vi "Make DIO JSON.vi"(9 "Force":bool, 10 "DIO prev":T1={"type"="DIO", "device"="", "name"="", "data"={"<init"=FALSE, "<>value"=FALSE, "<pulse_length"=0, "<input"=FALSE}}, 11 "DIO new":T1={"type"="DIO", "device"="", "name"="", "data"={"<init"=FALSE, "<>value"=FALSE, "<pulse_length"=0, "<input"=FALSE}}) -> (3 "delta JSON":string)   [LabVIEW 2019]
uses:
  DIO data proto.ctl
  DIO proto.ctl
panel:
  out "Complete JSON":string
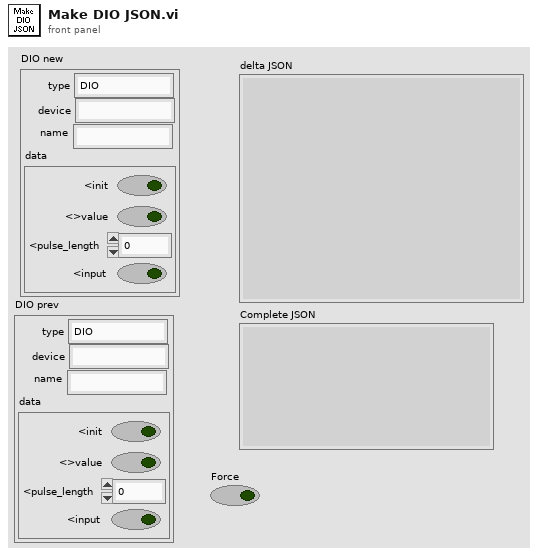
[diagram p1: front panel]
types:
  T1 = typedef "DIO proto.ctl" = cluster{"type":string, "device":string, "name":string, "data":T2}
  T2 = typedef "DIO data proto.ctl" = cluster{"<init":bool, "<>value":bool, "<pulse_length":i32, "<input":bool}
  T3 = cluster{"type":bool, "device":bool, "name":bool, "data":cluster{"<init":bool, "<>value":bool, "<pulse_length":bool, "<input":bool}}
  T4 = cluster{"<init":bool, "<>value":bool, "<pulse_length":bool, "<input":bool}
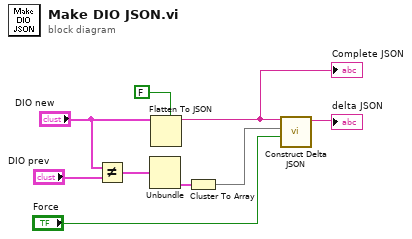
[diagram p0: block diagram]
diagram:
  n1 = Not Equal?(x="DIO new", y="DIO prev") -> (x != y?=w1:T3)
  n2 = Unbundle(w1) -> ("data"=w6:T4)  [unwired: 3 out]
  n3 = Flatten To JSON(enable LabVIEW extensions? (T)=FALSE, anything="DIO new") -> (JSON string=w5:string)  [unwired: 1 in, 1 out]
  "Complete JSON" <- w5
  n4 = Cluster To Array(cluster=w6) -> (array=w3:bool[])
  n5 = call "Construct Delta JSON.vi"("Force"="Force", "Checked Items"=w3, "JSON string"=w5) -> ("Delta JSON"=→"delta JSON":string)  [unwired: 8 in]
